vi "Get DAQ Device Information.vi"(8 "error in (no error)":errorcluster, 10 "information type":u32(ring) items=["NI-DAQ version", "device name", "base address", "data transfer mode for analog input", "data transfer mode for analog output group 1", "data transfer mode for analog output group 2", "data transfer mode for GPCTR 0", "data transfer mode for GPCTR 1", "data transfer mode for digital I/O group 1", "data transfer mode for digital I/O group 2", "device type code", "DMA A level", "DMA B level", "DMA C level", "interrupt A level", "interrupt B level", "reserved", "lpt device mode", "DAQCard-700 counter 1 source", "interrupt generation mode", "device state during suspend mode", "computer name", "serial number", "counter type", "Scarab A Memory Size", "Scarab B Memory Size"], 11 "task ID or device":u32 format="%.0x") -> (0 "error out":errorcluster, 2 "information string":string, 3 "task ID out":u32 format="%.0x")   [LabVIEW 2013]
doc: "Returns information about a DAQ device."
uses:
  <vilib>/DAQ/lvdaq.dll
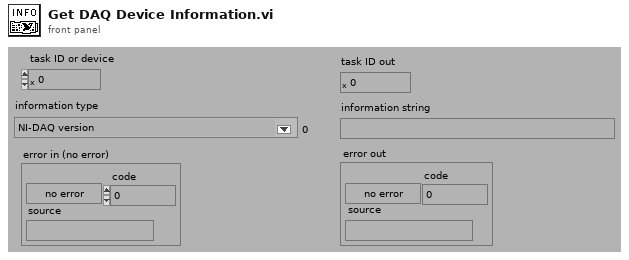
[diagram p1: front panel]
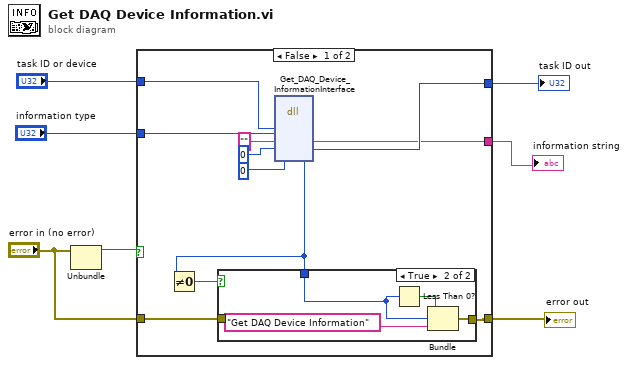
[diagram p0: block diagram]
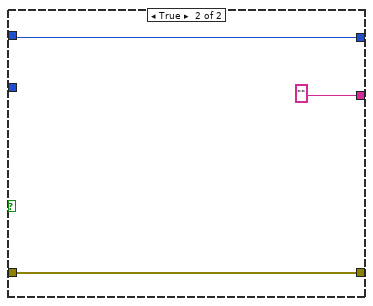
[diagram p3: hidden frame]
diagram:
  n1 = Unbundle("error in (no error)") -> ("status"=w7:bool)  [unwired: 2 out]
  n2 = case shown="False" w7 {
    tunnel: "error in (no error)" -> [w18 w26]
    tunnel: [w17 w26] -> w5
    tunnel: "task ID or device" -> [w10 w25]
    tunnel: [w13 w25] -> w3
    tunnel: [w12 ""] -> w2
    tunnel: "information type" -> [w11 _]
    frame False {
      n3 = dll-call lib="C:/Program Files/National Instruments/LabVIEW 7.1/vi.lib/DAQ/lvdaq.dll" fn="Get_DAQ_Device_InformationInterface"("task ID or device"=w10, "information type"=w11, "", u32 0, 0) -> (w12:string, w13:u32, w8:i32)  [unwired: 6 in, 2 out]
      n4 = Not Equal To 0?(x=w8) -> (x != 0?=w16:bool)
      n5 = case shown="True" w16 {
        tunnel: w18 -> [w19 _]
        tunnel: [w19 w20] -> w17
        tunnel: w8 -> [_ w21]
        frame False {
        }
        frame True {
          n6 = Less Than 0?(x=w21) -> (x < 0?=w22:bool)
          n7 = Bundle(w22, w21, "Get DAQ Device Information") -> (w20:errorcluster)  [unwired: 1 in]
        }
      }
    }
    frame True {
    }
  }
  "task ID out" <- w3
  "error out" <- w5
  "information string" <- w2
